vi "is Integer.vi"(11 "<JSON>":string) -> (3 "is Integer?":bool)   [LabVIEW 2017, in "JSONtext.lvlib"]
uses:
  JSONtext.lvlib
  <vilib>/regexp/Match Regular Expression.xnode
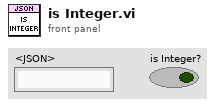
[diagram p1: front panel]
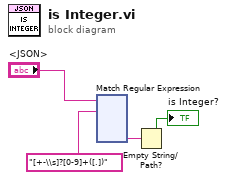
[diagram p0: block diagram]
diagram:
  n1 = xnode "Match Regular Expression"("input string"="<JSON>", "regular expression"="[+-\\s]?[0-9]+([.])") -> ("submatch 1"=w1:string)  [unwired: 4 in, 5 out]
  n2 = Empty String/Path?(string/path=w1) -> (empty?=→"is Integer?":bool)
